vi "GET.vi"(6 "timeout":i32=10000, 7 "output file":path, 8 "error in":errorcluster, 10 "url":string, 11 "http-method in":refnum<class "REST Client.lvclass">) -> (0 "error out":errorcluster, 2 "response":refnum<class "response.lvclass">, 3 "http-method out":refnum<class "REST Client.lvclass">)   [LabVIEW 2020, in "REST Client.lvlib" / "REST Client.lvclass"]
uses:
  REST Client.lvclass
  response/response.lvclass
  http-client/http-client.lvclass
  REST Client.lvclass/REST Client.ctl
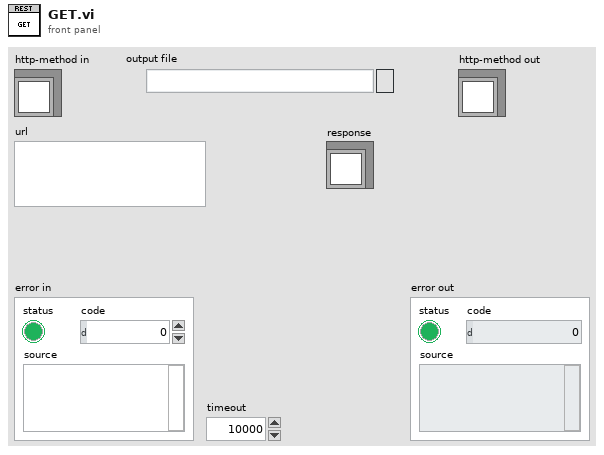
[diagram p1: front panel]
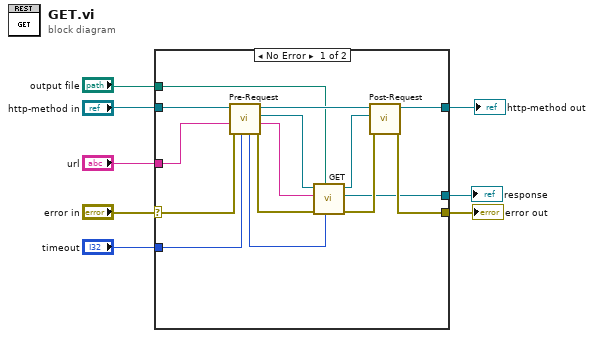
[diagram p0: block diagram]
diagram:
  n1 = case shown="No Error" "error in" {
    selector: "error in" -> [w20 w25]
    tunnel: [w17 w25] -> w6
    tunnel: [w18 w24] -> w5
    tunnel: "http-method in" -> [w19 w24]
    tunnel: "url" -> [w9 _]
    tunnel: "timeout" -> [w12 _]
    tunnel: [w16 _] -> w7
    tunnel: "output file" -> [w15 _]
    frame No Error {
      n2 = call "Pre-Request.vi"("timeout"=w12, "error in (no error)"=w20, "url"=w9, "REST Client in"=w19) -> ("error out"=w22:errorcluster, "Resolved URL"=w10:string, "http-client"=w14:refnum<class "http-client.lvclass">, "REST Client out"=w23:refnum<class "REST Client.lvclass">, "Timeout"=w11:i32)  [unwired: 3 in]
      n3 = call-dynamic "GET.vi"("timeout"=w11, "output file"=w15, "error in"=w22, "url"=w10, "http-method in"=w14) -> ("error out"=w21:errorcluster, "response"=w16:refnum<class "response.lvclass">, "http-method out"=w13:refnum<class "http-client.lvclass">)  [unwired: 4 in]
      n4 = call "Post-Request.vi"("error in (no error)"=w21, "http-method in"=w13, "REST Client in"=w23) -> ("error out"=w17:errorcluster, "REST Client out"=w18:refnum<class "REST Client.lvclass">)  [unwired: 7 in]
    }
    frame Error {
    }
  }
  "error out" <- w6
  "http-method out" <- w5
  "response" <- w7
